vi "cook.vi"(8 "error in (no error)":errorcluster, 11 "Toaster in":refnum<class "Toaster.lvclass">) -> (0 "error out":errorcluster, 3 "Toaster out":refnum<class "Toaster.lvclass">)   [LabVIEW 2010, in "Toaster.lvclass"]
uses:
  Toaster.lvclass
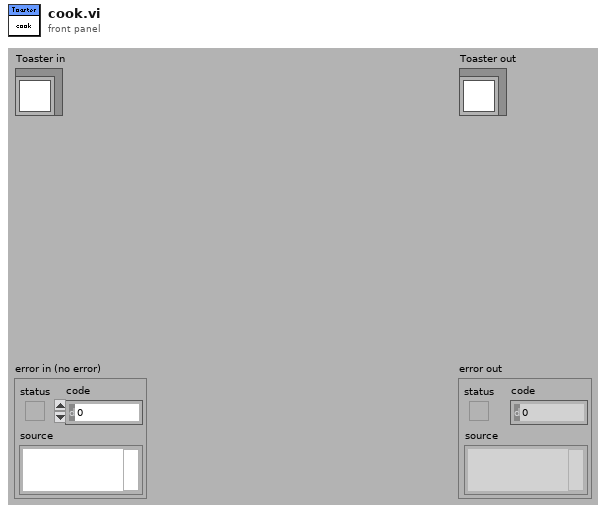
[diagram p1: front panel]
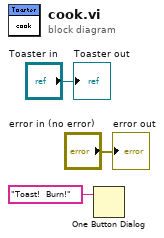
[diagram p0: block diagram]
diagram:
  n1 = One Button Dialog(message="Toast!  Burn!") -> ()  [unwired: 1 in, 1 out]
  "error out" <- "error in (no error)"
  "Toaster out" <- "Toaster in"
